vi "Teleop.vi"(10 "Match Info":T1={"Autonomous Elapsed Seconds"=0.0, "TeleOp Elapsed Seconds"=0.0, "Disabled Elapsed Seconds"=0.0, "Visited Autonomous"=FALSE, "Visited TeleOp"=FALSE, "Visited Disabled"=FALSE, "Autonomous Settings"={"Autonomous Style"=enum."Independent", "VI Refnum"=refnum}}, 11 "Call Context":T2) -> ()   [LabVIEW 2014]
doc: "This VI is called for each TeleOp packet received from the DS where the robot is not disabled. It is often used to read from the joysticks and update I/O or to update setpoints for timed control loops. It should complete and return within 20 milliseconds or it may miss DS packets."
uses:
  <vilib>/Rock Robotics/WPI/DriverStation/WPI_DriverStationDerivedRobotMode.ctl
  <vilib>/Rock Robotics/WPI/DriverStation/WPI_DriverStationMatch Info.ctl
  <vilib>/Rock Robotics/Network Tables/SD Read Boolean.vi
  <vilib>/Rock Robotics/Network Tables/SD Read Number.vi
  <vilib>/Rock Robotics/WPI/Ultrasonic/WPI_SonarMB1010AnalogRefNum Registry Get.vi
  <vilib>/Rock Robotics/WPI/Ultrasonic/WPI_SonarMB1010AnalogGetRange.vi
  Robot Global Data.vi
panel:
  out "Angle 2":dbl
  out "Distance 2":dbl
  out "Distance":dbl
  out "Angle":dbl
  out "Sample Slider 0":dbl(slide) scale=0.0..5.0
  out "Sample Boolean 1":bool
  out "Sample Boolean 0":bool
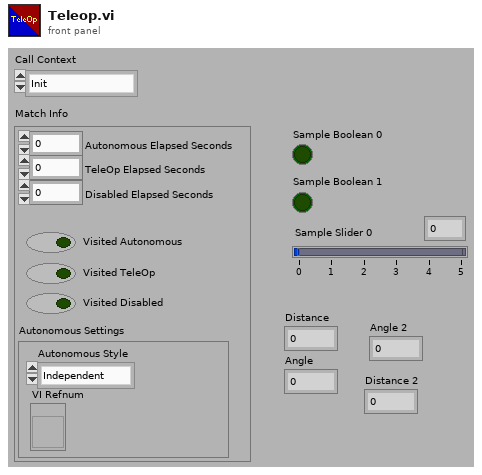
[diagram p1: front panel]
types:
  T1 = typedef "WPI_DriverStationMatch Info.ctl" = cluster{"Autonomous Elapsed Seconds":dbl, "TeleOp Elapsed Seconds":dbl, "Disabled Elapsed Seconds":dbl, "Visited Autonomous":bool, "Visited TeleOp":bool, "Visited Disabled":bool, "Autonomous Settings":cluster{"Autonomous Style":enum16{"Iterative", "Independent"}, "VI Refnum":refnum<vi>}}
  T2 = typedef "WPI_DriverStationDerivedRobotMode.ctl" = enum16{"Init", "Execute", "Stop"}
  T3 = typedef "WPI_GyroDevRef.ctl" = cluster{"DevStatus":errorcluster, "Analog Module":T4, "Analog Channel":T5, "Offset":dbl, "Gain (VoltsPerDegree/Second)":dbl}
  T4 = typedef "FPGA_TypedefAnalogModule.ctl" = enum16{"Controller 1"}
  T5 = typedef "FPGA_AIChannel.ctl" = enum8{"AI 0", "AI 1", "AI 2", "AI 3", "AI MXP 0", "AI MXP 1", "AI MXP 2", "AI MXP 3", "Invalid"}
  T6 = typedef "WPI_SonarMB1010AnalogDeviceRef.ctl" = cluster{"AIDeviceRef":T7, "Scaling factor (V/in)":dbl, "Average Bits":u8}
  T7 = typedef "WPI_AnalogChannelDevRef.ctl" = cluster{"DevStatus":errorcluster, "Controller":T4, "Analog Channel":T5}
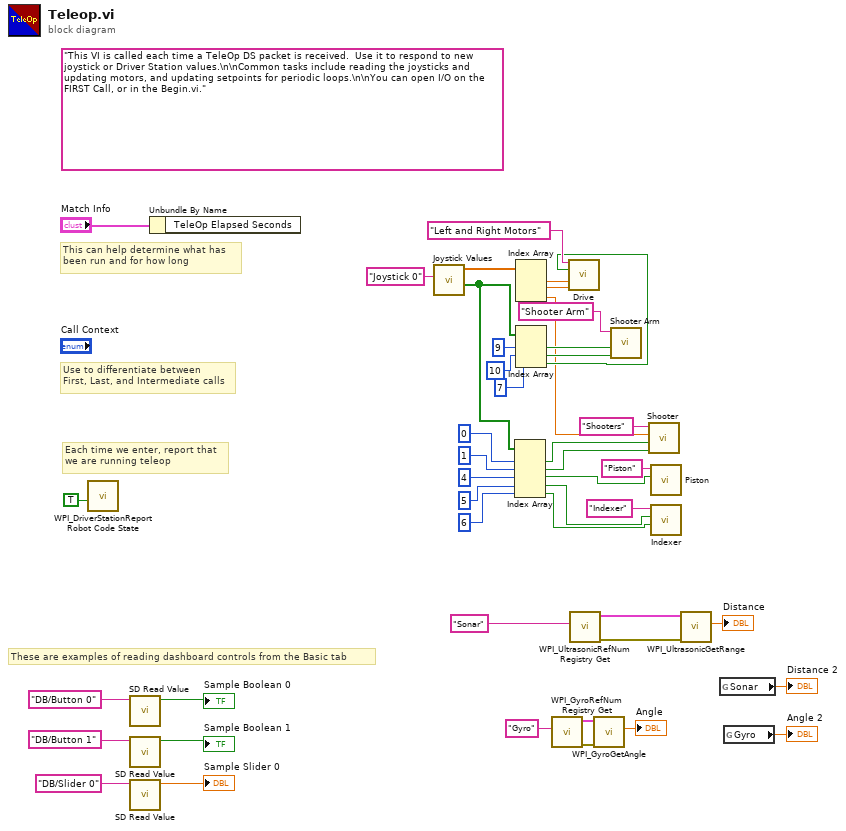
[diagram p0: block diagram]
diagram:
  (unwired) "This VI is called each time a TeleOp DS packet is received.  Use it to respond to new joystick or Driver Station values.\n\nCommon tasks include reading the joysticks and updating motors, and updating setpoints for periodic loops.\n\nYou can open I/O on the FIRST Call, or in the Begin.vi."
  # "These are examples of reading dashboard controls from the Basic tab"
  # "Each time we enter, report that\nwe are running teleop"
  # "Use to differentiate between\nFirst, Last, and Intermediate calls"
  # "This can help determine what has\nbeen run and for how long"
  n1 = call <vilib>:"WPI_DriverStationReport Robot Code State.vi"("TeleOp"=TRUE ("Autonomous")) -> ()  [unwired: 10 in, 1 out]
  n2 = call-poly <vilib>:"SD Read Value.vi"("Name"="DB/Button 0" ("refnum name")) -> ("Boolean"=→"Sample Boolean 0":bool)  [unwired: 8 in, 2 out]
  n3 = call-poly <vilib>:"SD Read Value.vi"("Name"="DB/Button 1" ("refnum name")) -> ("Boolean"=→"Sample Boolean 1":bool)  [unwired: 8 in, 2 out]
  n4 = call-poly <vilib>:"SD Read Value.vi"("Name"="DB/Slider 0" ("refnum name")) -> ("Numeric"=→"Sample Slider 0":dbl)  [unwired: 8 in, 2 out]
  n5 = Unbundle By Name("Match Info") -> ()  [unwired: 1 out]
  n6 = call "Joystick Values.vi"("Joystick Ref"="Joystick 0") -> ("Buttons"=w23:bool[], "Axes"=w12:dbl[])  [unwired: 9 in]
  n7 = Index Array(array=w23, index #1=0 ("index"), index #2=1 ("index"), index #3=4 ("index"), index #4=5 ("index"), index #5=6 ("index")) -> (element #1=w21:bool, element #2=w20:bool, element #3=w18:bool, element #4=w16:bool, element #5=w15:bool)
  n8 = Index Array(array=w12) -> (element #1=w36:dbl, element #2=w35:dbl, element #3=w11:dbl)  [unwired: 3 in]
  n9 = Index Array(array=w23, index #1=9 ("index"), index #2=10 ("index"), index #3=7 ("index")) -> (element #1=w31:bool, element #2=w30:bool, element #3=w13:bool)
  n10 = call <vilib>:"WPI_GyroRefNum Registry Get.vi"("refnum name"="Gyro") -> ("error out"=w4:errorcluster, "GyroDevRef"=w5:T3)  [unwired: 9 in]
  n11 = call "Drive.vi"("Motor Ref"="Left and Right Motors" ("refnum name"), "Boolean"=w13, "X"=w36, "Y"=w35) -> ()  [unwired: 12 in]
  n12 = call-poly <vilib>:"WPI_UltrasonicRefNum Registry Get.vi"("refnum name"="Sonar") -> ("error out"=w7:errorcluster, "SonarMB1010AnalogDevRef"=w8:T6)  [unwired: 9 in]
  n13 = call <vilib>:"WPI_GyroGetAngle.vi"("error in (no error)"=w4, "GyroDevRef"=w5) -> ("Angle"=→"Angle":dbl)  [unwired: 6 in, 3 out]
  n14 = call "Shooter Arm.vi"("Boolean 2"=w30, "Boolean"=w31, "Arm Ref"="Shooter Arm" ("refnum name")) -> ()  [unwired: 9 in]
  n15 = call "Shooter.vi"("Boolean 2"=w20, "Boolean"=w21, "Power"=w11, "Motor Ref"="Shooters") -> ()  [unwired: 8 in]
  n16 = call "Piston.vi"("Boolean"=w18, "refnum name"="Piston") -> ()  [unwired: 10 in]
  n17 = call "Indexer.vi"("Boolean 2"=w15, "Boolean"=w16, "refnum name"="Indexer") -> ()  [unwired: 9 in]
  n18 = call-poly <vilib>:"WPI_UltrasonicGetRange.vi"("error in"=w7, "SonarMB1010AnalogDevRef"=w8) -> ("Distance"=→"Distance":dbl)  [unwired: 7 in, 2 out]
  n19 = global read "Robot Global Data.vi" "Sonar"() -> (→"Distance 2":dbl)
  n20 = global read "Robot Global Data.vi" "Gyro"() -> (→"Angle 2":dbl)
